vi "DIAG_STM Get Connection Reference.vi"   [LabVIEW 2015, in "Diagnostics Addon Engine.lvlib"]
doc: "Returns the connection reference of the STM session."
uses:
  Diagnostics Addon Engine.lvlib
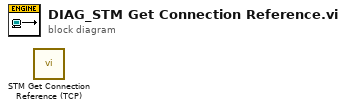
[diagram p0: block diagram]
diagram:
  n1 = call "STM Get Connection Reference (TCP).vi"() -> ()  [unwired: 9 in, 3 out]
